vi "ROM Diagnostics.vi"() -> (0 "error out":errorcluster, 3 "Result":bool)   [LabVIEW 2011]
doc: "Performs diagnostics on the Read Only Memory (ROM) on the motherboard."
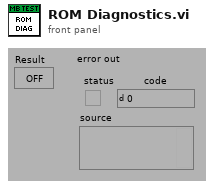
[diagram p1: front panel]
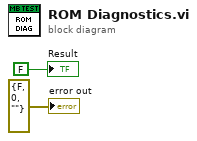
[diagram p0: block diagram]
diagram:
  "error out" <- errorcluster {"status"=FALSE, "code"=0, "source"=""} ("error out")
  "Result" <- FALSE ("PASS/FAIL Flag")
